vi "Coral Target Loop.vi"(0 "Camera Name":string="cam0") -> ()   [LabVIEW 2025]
uses:
  <vilib>/Utility/config.llb/NI_LVConfig.lvlib
  <vilib>/Utility/config.llb/Write Key (String).vi
  <vilib>/vision/NI_Vision_Development_Module.lvlib
  Camera Set Up/Event/Event Setup Types.ctl
  Ball/State Machine/Ball States.ctl
  <vilib>/Utility/config.llb/Read Key (String).vi
  Steam Type.ctl
  State Machine/Coral States.ctl
  <vilib>/vision/Image Controls.llb/IMAQ Image.ctl
  State Machine/Coral Main CLuster.ctl
  <vilib>/Rock Robotics/Network Tables/NT Write String.vi
  April Tags/Camera Info.ctl
panel:
  in  "Main":enum32{"Page 1", "Page 2"}(tab)
  out "Algae Distance":dbl[](array[numeric]) caption="Distance" format="%.1f"
  out "Algae Angle":dbl[](array[numeric]) caption="Angle" format="%.1f"
  out "Image":T1(plugin-control)
  in  "Settings":bool
  in  "Save":bool
  in  "Tools":bool
  out "Ball Fps":dbl format="%#.0f"
  in  "Robot Calibration Cluster":T2={"Camera FOV Vert View Angle (deg)"=34.5, "Camera FOV Hor View Angle (deg)"=28.3, "Distance Correction Factor"=0.946} {"Distance Correction Factor" format="%#_13g"; "Camera FOV Hor View Angle (deg)" format="%#_13g"; "Camera FOV Vert View Angle (deg)" format="%#_13g"}
  in  "Home":bool
  in  "Coral Color Range":T3={"Hue"={21.620689392089844, 69.62068939208984}, "Sat"={66.41378784179688, 255.0}, "Val"={96.0, 255.0}} caption="Color Range" {"Hue" scale=0.0..255.0 scale format="%#_3g"}
  out "Mask":T1(plugin-control)
  in  "Score Threshold %":dbl=80.0
  # "Edit the camera name to the camera that you are going to use for this target package"
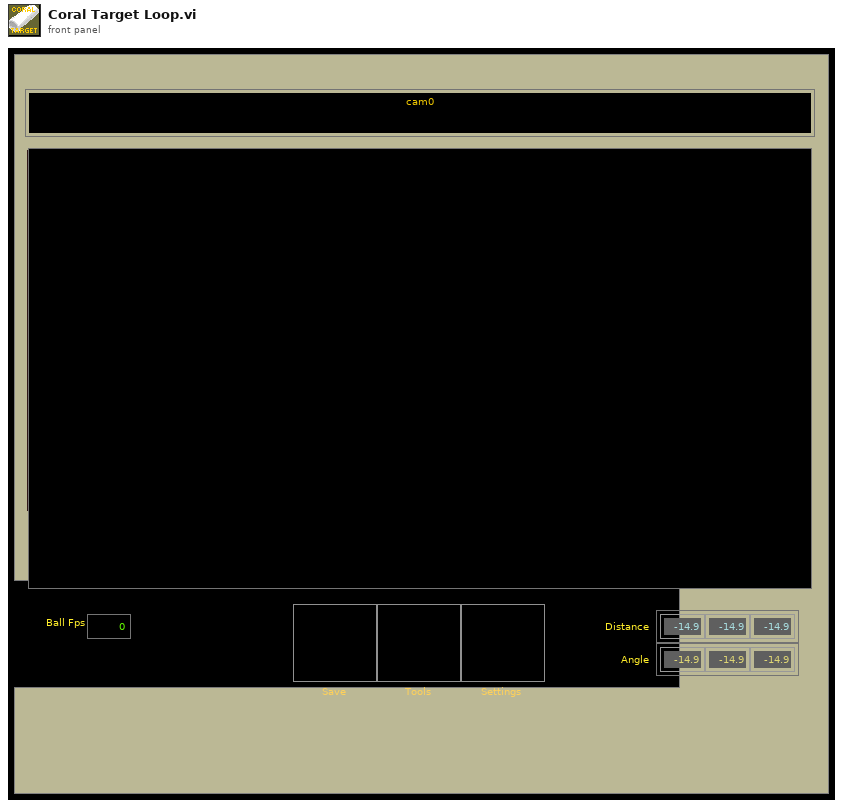
[diagram p1: front panel]
types:
  T1 = typedef "IMAQ Image.ctl" = refnum<image>
  T2 = typedef "Camera Info.ctl" = cluster{"Camera FOV Vert View Angle (deg)":dbl, "Camera FOV Hor View Angle (deg)":dbl, "Distance Correction Factor":dbl}
  T3 = cluster{"Hue":cluster{dbl, dbl}, "Sat":cluster{dbl, dbl}, "Val":cluster{dbl, dbl}}
  T4 = typedef "Coral Main CLuster.ctl" = cluster{"Coral FIFO":T5[], "Camera Name":string, "Coral path":path, "Control Ref's":refnum<vi>[], "Greyscale Mask Image":T1, "Main Image":T1, "Coral Color Range":cluster{"Hue":cluster{dbl, dbl}, "Sat":cluster{dbl, dbl}, "Val":cluster{dbl, dbl}}, "Timeout":i32}
  T5 = typedef "Coral States.ctl" = enum16{"Message Dispatcher", "INI", "Open", "Save", "Exit"}
  T6 = typedef "Particle Parameters" = i32
  T7 = typedef "Steam Type.ctl" = enum8{"Unknown", "Apriltag", "Algae", "Coral"}
  T8 = typedef "Event Setup Types.ctl" = enum16{"Default", "Camera Loop Started", "Close Settings", "GreyScale", "Open Front Panel", "Reset Team Number", "Save Data", "Exit"}
  T9 = typedef "Ball States.ctl" = enum16{"Message Dispatcher", "INI", "Open", "Save", "Exit"}
  T10 = typedef "Target Fields.ctl" = cluster{"diameter points":cluster{"first point":cluster{"x":dbl, "y":dbl}, "projected point":cluster{"x":dbl, "y":dbl}}, "normalized center":cluster{"x":dbl, "y":dbl}, "Overall Score":dbl, "Area Score":dbl, "Moment Score":dbl, "Aspect Score":dbl, "Distance (ft)":dbl, "Upper Goal":bool}
  T11 = typedef "Event Setup Types.ctl" = enum16{"Default", "Camera Loop Started", "GreyScale", "Reset Camera Settings", "Reset Team Number", "Save Data", "Setting Changed", "Update Video Mode", "Video Mode Changed", "Exit"}
  T12 = cluster{cluster{"Lower":dbl, "Upper":dbl}, cluster{"Lower":dbl, "Upper":dbl}, cluster{"Lower":dbl, "Upper":dbl}}
  T13 = typedef "Image Type" = u32
  T14 = typedef "NI_LVConfig.lvlib/Config Data RefNum.ctl" = refnum<k1>
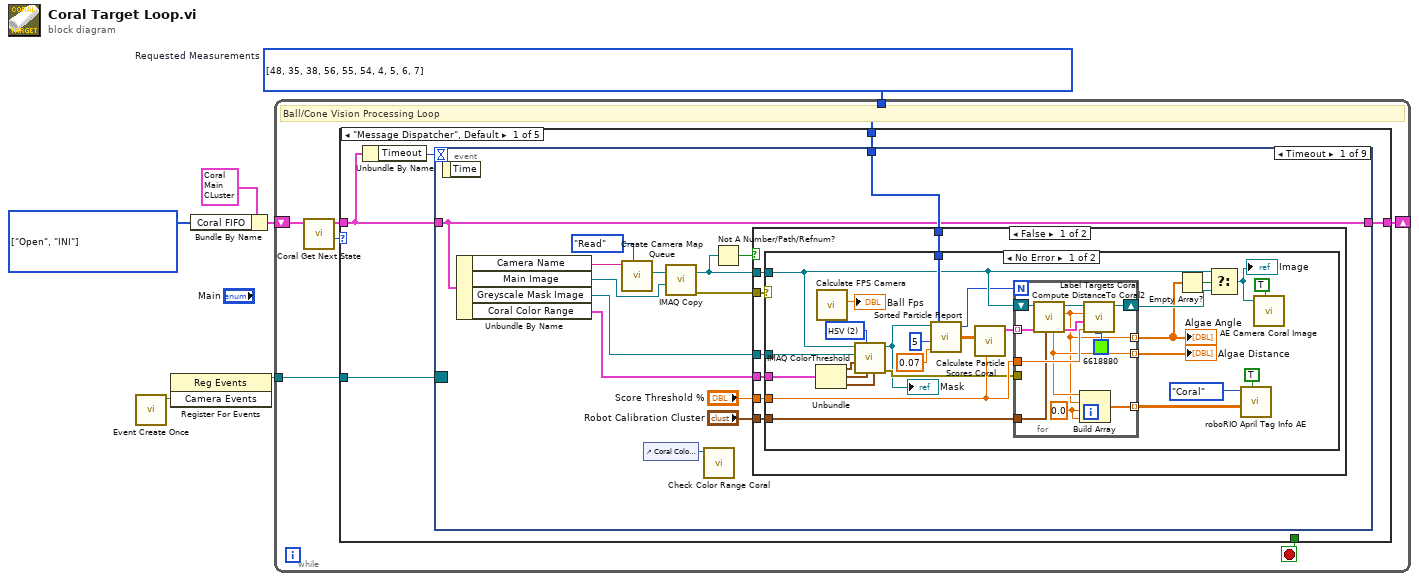
[diagram p0: block diagram]
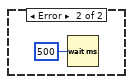
[diagram p2: hidden frame]
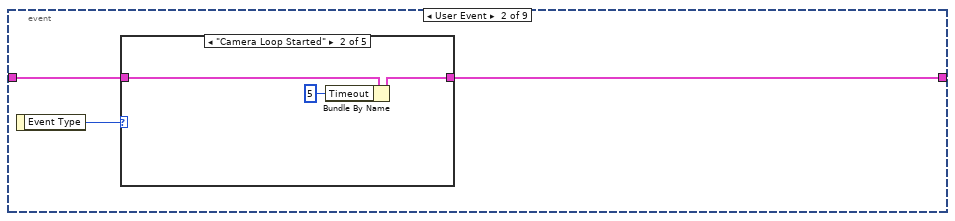
[diagram p4: hidden frame]
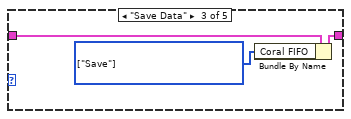
[diagram p6: hidden frame]
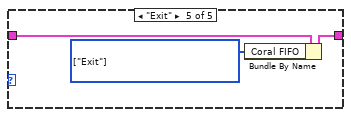
[diagram p8: hidden frame]
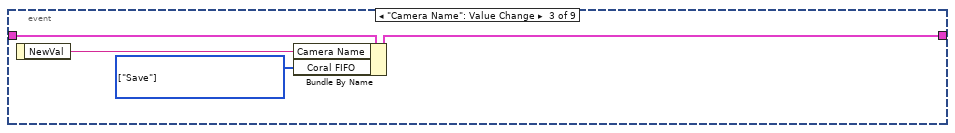
[diagram p9: hidden frame]
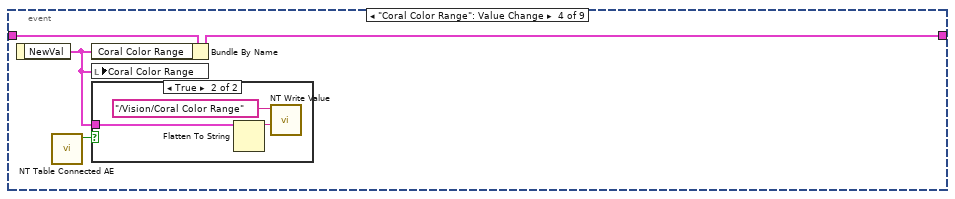
[diagram p10: hidden frame]
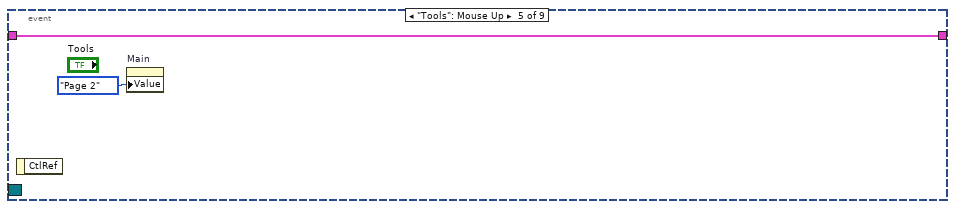
[diagram p12: hidden frame]
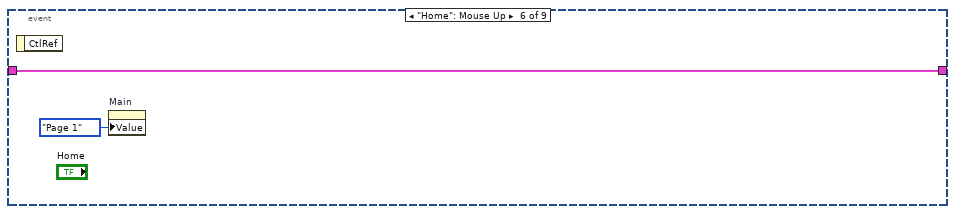
[diagram p13: hidden frame]
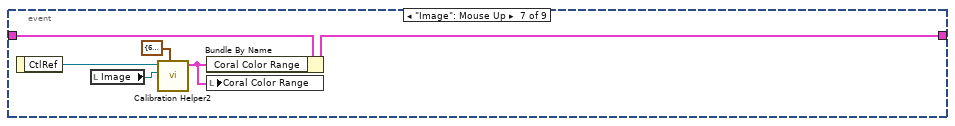
[diagram p14: hidden frame]
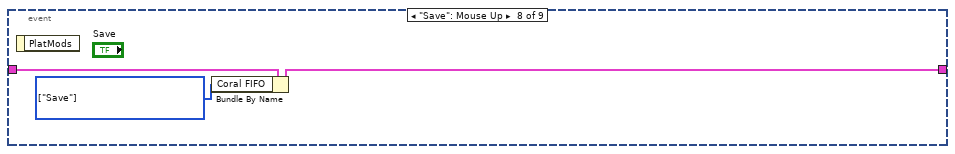
[diagram p15: hidden frame]
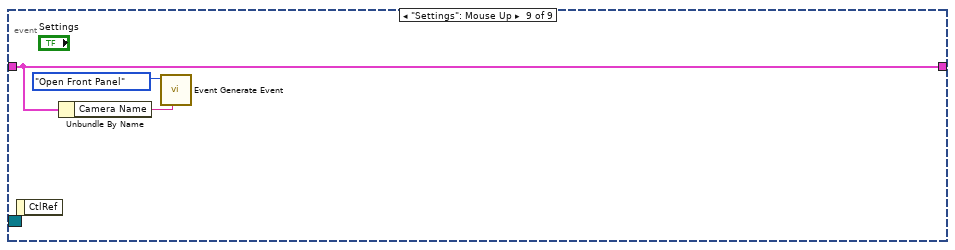
[diagram p16: hidden frame]
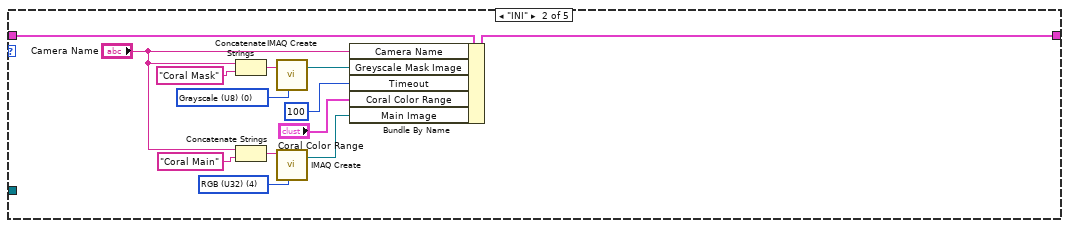
[diagram p17: hidden frame]
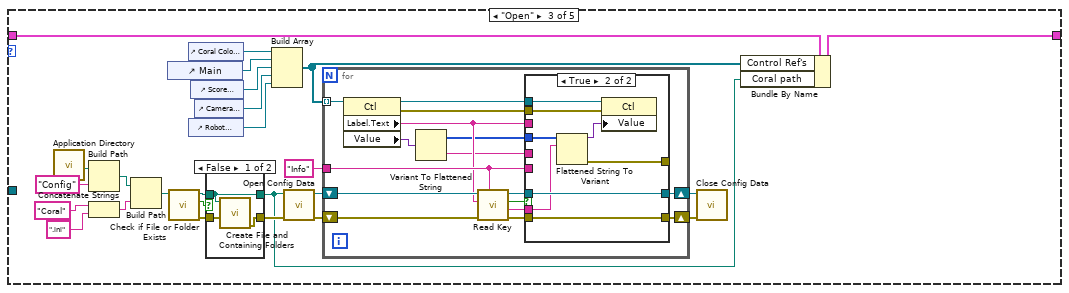
[diagram p18: hidden frame]
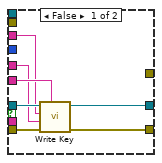
[diagram p20: hidden frame]
diagram:
  w2 = T5[] [enum."Open", enum."INI"] items=["Message Dispatcher", "INI", "Open", "Save", "Exit"] ("Ball FIFO")
  w4 = T6[] [48, 35, 38, 56, 55, 54, 4, 5, 6, 7] items=["Center of Mass X", "Center of Mass Y", "First Pixel X", "First Pixel Y", "Bounding Rect Left", "Bounding Rect Top", "Bounding Rect Right", "Bounding Rect Bottom", "Max Feret Diameter Start X", "Max Feret Diameter Start Y", "Max Feret Diameter End X", "Max Feret Diameter End Y", "Max Horiz. Segment Length Left", "Max Horiz. Segment Length Right", "Max Horiz. Segment Length Row", "-", "Bounding Rect Width", "Bounding Rect Height", "Bounding Rect Diagonal", "Perimeter", "Convex Hull Perimeter", "Holes' Perimeter", "Max Feret Diameter", "Equivalent Ellipse Major Axis", "Equivalent Ellipse Minor Axis", "Equivalent Ellipse Minor Axis (Feret)", "Equivalent Rect Long Side", "Equivalent Rect Short Side", "Equivalent Rect Diagonal", "Equivalent Rect Short Side (Feret)", "Average Horiz. Segment Length", "Average Vert. Segment Length", "Hydraulic Radius", "Waddel Disk Diameter", "-", "Area", "Holes' Area", "Particle & Holes' Area", "Convex Hull Area", "Image Area", "-", "Number of Holes", "Number of Horiz. Segments", "Number of Vert. Segments", "-", "Orientation", "Max Feret Diameter Orientation", "-", "% Area/Image Area", "% Area/(Particle & Holes' Area)", "Ratio of Equivalent Ellipse Axes", "Ratio of Equivalent Rect Sides", "-", "Elongation Factor", "Compactness Factor", "Heywood Circularity Factor", "Type Factor", "-", "Sum X", "Sum Y", "Sum XX", "Sum XY", "Sum YY", "Sum XXX", "Sum XXY", "Sum XYY", "Sum YYY", "-", "Moment of Inertia XX", "Moment of Inertia XY", "Moment of Inertia YY", "Moment of Inertia XXX", "Moment of Inertia XXY", "Moment of Inertia XYY", "Moment of Inertia YYY", "Norm. Moment of Inertia XX", "Norm. Moment of Inertia XY", "Norm. Moment of Inertia YY", "Norm. Moment of Inertia XXX", "Norm. Moment of Inertia XXY", "Norm. Moment of Inertia XYY", "Norm. Moment of Inertia YYY", "Hu Moment 1", "Hu Moment 2", "Hu Moment 3", "Hu Moment 4", "Hu Moment 5", "Hu Moment 6", "Hu Moment 7"]  # Requested Measurements
  n1 = call "Event Create Once.vi"() -> ("Camera Events"=w6:refnum<user-event>)  [unwired: 10 in, 1 out]
  n2 = register-events(w6) -> (reference out=w5:refnum<event-registration>)  [unwired: 2 in, 1 out]
  n3 = Bundle By Name(cluster=T4 {"Coral FIFO"=[], "Camera Name"="", "Coral path"=path "", "Control Ref's"=[], "Greyscale Mask Image"=refnum, "Main Image"=refnum, "Coral Color Range"={"Hue"={21.620689392089844, 69.62068939208984}, "Sat"={66.41378784179688, 255.0}, "Val"={96.0, 255.0}}, "Timeout"=5} ("output cluster"), "Coral FIFO"=w2) -> (w3:T4)
  n4 = while {
    tunnel: w4 -> [w13]
    tunnel: w5 -> [w12]
    shift-right: [w7] -> _
    shift-left: w3 -> [w10]
    stop <- w11 stop-if-true
    # "Ball/Cone Vision Processing Loop"
    n5 = call "Coral Get Next State.vi"("Coral Main Cluster in"=w10) -> ("Next State"=w9:T9, "Coral Main Cluster out"=w8:T4)  [unwired: 9 in]
    n6 = case shown="\"Message Dispatcher\", Default" w9 {
      tunnel: w13 -> [w18 _ _ _ _]
      tunnel: w12 -> [w17 _ _ _ _]
      tunnel: [_ _ _ _ TRUE] -> w11
      tunnel: w8 -> [w15 w130 w144 w197 w214]
      tunnel: [w16 w129 w142 w197 w214] -> w7
      frame "Message Dispatcher", Default {
        n7 = Unbundle By Name(w15) -> ("Timeout"=w14:i32)
        n8 = event shown="[0] Timeout" {
          selector: w17 -> [_ _ _ _ _ _ _ _ _]
          dyn-events: _ -> [_ _ _ _ _ _ _ _ _]
          timeout: w14 -> [_ _ _ _ _ _ _ _ _]
          tunnel: w18 -> [w32 _ _ _ _ _ _ _ _]
          tunnel: w15 -> [w27 w82 w97 w101 w105 w107 w111 w117 w119]
          tunnel: [w27 w80 w96 w100 w105 w107 w110 w116 w119] -> w16
          event Timeout {
            n9 = event-data() -> ()  [unwired: 1 in, 1 out]
            n10 = Unbundle By Name(w27) -> ("Camera Name"=w29:string, "Main Image"=w24:T1, "Greyscale Mask Image"=w28:T1, "Coral Color Range"=w26:T3)
            n11 = call "Create Camera Map Queue.vi"("Action"=enum16{"Read", "Write"}."Read", "Camera"=w29) -> ("Image out"=w25:T1)  [unwired: 8 in, 1 out]
            n12 = control-ref of="Coral Color Range"() -> (w21:refnum<vi>)
            n13 = call "IMAQ Copy"("Image Dst"=w24, "Image Src"=w25) -> ("error out"=w23:errorcluster, "Image Dst Out"=w19:T1)  [unwired: 4 in]
            n14 = call "Check Color Range Coral.vi"("Coral Color Range"=w21) -> ()  [unwired: 11 in]
            n15 = Not A Number/Path/Refnum?(number/path/refnum=w19) -> (NaN/Path/Refnum?=w20:bool)
            n16 = case shown="False" w20 {
              tunnel: w32 -> [w39 _]
              tunnel: "Score Threshold %" -> [w38 _]
              tunnel: w28 -> [w37 _]
              tunnel: w26 -> [w36 _]
              tunnel: w19 -> [w35 _]
              tunnel: w23 -> [w34 _]
              tunnel: "Robot Calibration Cluster" -> [w33 _]
              frame False {
                n17 = case shown="No Error" w34 {
                  tunnel: w39 -> [w66 _]
                  tunnel: w37 -> [w64 _]
                  tunnel: w36 -> [w63 _]
                  tunnel: w38 -> [w62 _]
                  tunnel: w35 -> [w61 _]
                  tunnel: w33 -> [w41 _]
                  frame No Error {
                    w56 = u16 2 items=["RGB", "HSL", "HSV", "HSI"] ("Color Mode")
                    n18 = Unbundle(w63) -> ("Hue"=w51:cluster{dbl, dbl}, "Sat"=w50:cluster{dbl, dbl}, "Val"=w49:cluster{dbl, dbl})
                    n19 = call "Calculate FPS Camera.vi"() -> ("Fps"=→"Ball Fps":dbl)  [unwired: 11 in]
                    n20 = call "IMAQ ColorThreshold"("Blue or Luma or Val or Inten Range"=w49, "Green or Sat Range"=w50, "Color Mode"=w56, "Red or Hue Range"=w51, "Image Dst"=w64, "Image Src"=w61) -> ("error out"=w55:errorcluster, "Image Dst Out"=w40:T1)  [unwired: 4 in]
                    "Mask" <- w40
                    n21 = call "Sorted Particle Report.vi"("Min Area Size %"=0.07 ("Size Limit %"), "Particle Count Limit"=5 ("Particle Count LImit"), "Pixel Measurements"=w66, "Image in"=w40) -> ("Sorted Data"=w59:dbl[][], "Particles"=w54:i32)  [unwired: 1 out]
                    n22 = call "Calculate Particle Scores Coral.vi"("Limit"=w62, "Sorted Data"=w59) -> ("Scores"=w58:T10[])  [unwired: 9 in]
                    n23 = for {
                      N: w54 -> [_]
                      tunnel: w58 -> [w76] mode=indexing
                      shift-right: [w78] -> w53
                      shift-left: w61 -> [w74]
                      tunnel: w62 -> [w77]
                      tunnel: [w70] -> w48 mode=indexing
                      tunnel: w55 -> [_]
                      tunnel: [w71] -> w47 mode=indexing
                      tunnel: [w68] -> w42 mode=indexing
                      tunnel: w41 -> [w67]
                      w69 = 0.0 ("element")
                      n24 = call "Compute DistanceTo Coral2.vi"("Robot Calibration Cluster"=w67, "results 2"=w76, "Image Src"=w74) -> ("results out"=w73:T10, "Offset Angle"=w70:dbl, "Image Dst Out"=w75:T1, "Distance from target (in)"=w71:dbl)  [unwired: 5 in]
                      n25 = Build Array(w71, w70, w69, w69) -> (w68:dbl[])
                      n26 = call "Label Targets Coral.vi"("Color"=u32 6618880, "Score Threshold"=w77, "results"=w73, "Angle"=w70, "Image in"=w75) -> ("Image out"=w78:T1)  [unwired: 6 in]
                    }
                    "Algae Angle" <- w48
                    "Algae Distance" <- w47
                    n27 = Empty Array?(array=w48) -> (empty?=w52:bool)
                    n28 = Select(t=w61, s=w52, f=w53) -> (s? t:f=w65:T1)
                    "Image" <- w65
                    n29 = call "roboRIO April Tag Info AE.vi"("Update"=TRUE, "Info in"=w42, "Stream Type"=Steam_Type."Coral") -> ()  [unwired: 8 in, 1 out]
                    n30 = call "AE Camera Coral Image.vi"("Update"=TRUE, "Ball Image in"=w65) -> ()  [unwired: 9 in, 1 out]
                  }
                  frame Error {
                    n31 = Wait (ms)(milliseconds to wait=u32 500) -> ()  [unwired: 1 out]
                  }
                }
              }
              frame True {
              }
            }
          }
          event User Event {
            n32 = event-data() -> ("Event Type"=w81:T11)  [unwired: 1 in]
            n33 = case shown="\"Camera Loop Started\"" w81 {
              tunnel: w82 -> [w83 w86 w89 w90 w93]
              tunnel: [w83 w85 w88 w90 w92] -> w80
              frame "Default", Default {
              }
              frame "Camera Loop Started" {
                n34 = Bundle By Name(cluster=w86, "Timeout"=5) -> (w85:T4)
              }
              frame "Save Data" {
                w87 = T9[] [enum."Save"] items=["Message Dispatcher", "INI", "Open", "Save", "Exit"] ("Ball FIFO")
                n35 = Bundle By Name(cluster=w89, "Coral FIFO"=w87) -> (w88:T4)
              }
              frame "Default" {
              }
              frame "Exit" {
                w91 = T9[] [enum."Exit"] items=["Message Dispatcher", "INI", "Open", "Save", "Exit"] ("Ball FIFO")
                n36 = Bundle By Name(cluster=w93, "Coral FIFO"=w91) -> (w92:T4)
              }
            }
          }
          event "Camera Name": Value Change {
            w94 = T9[] [enum."Save"] items=["Message Dispatcher", "INI", "Open", "Save", "Exit"] ("Ball FIFO")
            n37 = event-data() -> ("NewVal"=w95:string)  [unwired: 1 in]
            n38 = Bundle By Name(cluster=w97, "Camera Name"=w95, "Coral FIFO"=w94) -> (w96:T4)
          }
          event "Coral Color Range": Value Change {
            n39 = event-data() -> ("NewVal"=w98:T3)  [unwired: 1 in]
            n40 = call "NT Table Connected AE.vi"() -> ("NT Table Connected out"=w99:bool)  [unwired: 11 in]
            n41 = Bundle By Name(cluster=w101, "Coral Color Range"=w98) -> (w100:T4)
            n42 = local write "Coral Color Range"(w98) -> ()
            n43 = case shown="True" w99 {
              tunnel: w98 -> [_ w102]
              frame False {
              }
              frame True {
                n44 = Flatten To String(anything=w102) -> (data string=w104:string)  [unwired: 3 in, 2 out]
                n45 = call-poly <vilib>:"NT Write Value.vi"("value"=w104, "name"="/Vision/Coral Color Range" ("Name")) -> ()  [unwired: 9 in, 1 out]
              }
            }
          }
          event "Tools": Mouse Up {
            n46 = event-data() -> ()  [unwired: 1 in, 1 out]
            n47 = property on="Main" class="TabCtl (strict)"("Value"=enum32{"Page 1", "Page 2"}."Page 2" ("Main")) -> ()  [unwired: 2 in, 2 out]
          }
          event "Home": Mouse Up {
            n48 = event-data() -> ()  [unwired: 1 in, 1 out]
            n49 = property on="Main" class="TabCtl (strict)"("Value"=enum32{"Page 1", "Page 2"}."Page 1" ("Main")) -> ()  [unwired: 2 in, 2 out]
          }
          event "Image": Mouse Up {
            n50 = event-data() -> ("CtlRef"=w113:refnum<vi>)  [unwired: 1 in]
            n51 = local read "Image"() -> (w112:T1)
            n52 = call "Calibration Helper2.vi"("Std Devs"=cluster{"H":dbl, "S":dbl, "V":dbl} {"H"=6.0, "S"=6.0, "V"=6.0} ("Std Devs Ball"), "Image"=w112, "Image Ctl Refnum"=w113) -> ("output color"=w109:T12)  [unwired: 7 in, 1 out]
            n53 = Bundle By Name(cluster=w111, "Coral Color Range"=w109) -> (w110:T4)
            n54 = local write "Coral Color Range"(w109) -> ()
          }
          event "Save": Mouse Up {
            w115 = T9[] [enum."Save"] items=["Message Dispatcher", "INI", "Open", "Save", "Exit"] ("Ball FIFO")
            n55 = event-data() -> ()  [unwired: 1 in, 1 out]
            n56 = Bundle By Name(cluster=w117, "Coral FIFO"=w115) -> (w116:T4)
          }
          event "Settings": Mouse Up {
            n57 = event-data() -> ()  [unwired: 1 in, 1 out]
            n58 = Unbundle By Name(w119) -> ("Camera Name"=w118:string)
            n59 = call "Event Generate Event.vi"("Camera Name"=w118, "Event Type"=Event_Setup_Types."Open Front Panel") -> ()  [unwired: 10 in]
          }
        }
      }
      frame "INI" {
        w126 = T13 4 items=["Grayscale (U8)", "Grayscale (I16)", "Grayscale (SGL)", "Complex (CSG)", "RGB (U32)", "HSL (U32)", "RGB (U64)", "Grayscale (U16)"] ("Image Type")
        w131 = T13 0 items=["Grayscale (U8)", "Grayscale (I16)", "Grayscale (SGL)", "Complex (CSG)", "RGB (U32)", "HSL (U32)", "RGB (U64)", "Grayscale (U16)"] ("Image Type")
        n60 = Concatenate Strings("Camera Name", "Coral Mask" ("string")) -> (w133:string)
        n61 = Concatenate Strings("Camera Name", "Coral Main" ("string")) -> (w125:string)
        n62 = call "IMAQ Create"("Image Name"=w133, "Image Type"=w131) -> ("New Image"=w128:T1)  [unwired: 2 in, 2 out]
        n63 = call "IMAQ Create"("Image Name"=w125, "Image Type"=w126) -> ("New Image"=w122:T1)  [unwired: 2 in, 2 out]
        n64 = Bundle By Name(cluster=w130, "Camera Name"="Camera Name", "Greyscale Mask Image"=w128, "Timeout"=100, "Coral Color Range"="Coral Color Range", "Main Image"=w122) -> (w129:T4)
      }
      frame "Open" {
        n65 = call <vilib>:"Application Directory.vi"() -> ("Application Directory"=w147:path)
        n66 = Build Path(base path=w147, name or relative path="Config") -> (appended path=w145:path)
        n67 = Concatenate Strings("Coral" ("string"), ".ini" ("name or relative path")) -> (w158:string)
        n68 = Build Path(base path=w145, name or relative path=w158) -> (appended path=w140:path)
        n69 = control-ref of="Main"() -> (w151:refnum<vi>)
        n70 = call <vilib>:"Check if File or Folder Exists.vi"("path"=w140) -> ("error out"=w136:errorcluster, "file or folder exists?"=w138:bool, "dup path"=w139:path)  [unwired: 8 in]
        n71 = control-ref of="Coral Color Range"() -> (w152:refnum<vi>)
        n72 = control-ref of="Robot Calibration Cluster"() -> (w134:refnum<vi>)
        n73 = control-ref of="Score Threshold %"() -> (w150:refnum<vi>)
        n74 = control-ref of="Camera Name"() -> (w135:refnum<vi>)
        n75 = case shown="False" w138 {
          tunnel: [w161 w162] -> w148
          tunnel: w139 -> [w160 w163]
          tunnel: [w160 w163] -> w137
          tunnel: w136 -> [w159 w162]
          frame False {
            n76 = call <vilib>:"Create File and Containing Folders.vi"("error in (no error)"=w159, "file path"=w160) -> ("error out"=w161:errorcluster)  [unwired: 8 in, 1 out]
          }
          frame True {
          }
        }
        n77 = Build Array(w152, w151, w150, w135, w134) -> (w141:refnum<vi>[])
        n78 = call <vilib>:"Open Config Data.vi"("error in (no error)"=w148, "configuration file path"=w137) -> ("error out"=w153:errorcluster, "refnum"=w157:T14)  [unwired: 7 in, 1 out]
        n79 = for {
          tunnel: "Info" ("Camera Name") -> [w176]
          tunnel: w141 -> [w166] mode=indexing
          shift-right: [w178] -> w156
          shift-left: w157 -> [w179]
          shift-right: [w177] -> w155
          shift-left: w153 -> [w175]
          n80 = property class="Ctl"(reference=w166) -> (reference out=w172:refnum<vi>, error out=w171:errorcluster, "Label.Text"=w169:string, "Value"=w165:variant)  [unwired: 1 in]
          n81 = Variant To Flattened String(Variant=w165) -> (data string=w167:string, 1:w164:i16[])
          n82 = call-poly <vilib>:"Read Key.vi"("section"=w176, "error in (no error)"=w175, "key"=w169, "refnum"=w179) -> ("error out"=w168:errorcluster, "value"=w173:string, "found?"=w174:bool, "refnum out"=w170:T14)  [unwired: 4 in]
          n83 = case shown="True" w174 {
            tunnel: w173 -> [_ w189]
            tunnel: w172 -> [_ w194]
            tunnel: w171 -> [_ w193]
            tunnel: w170 -> [w186 w192]
            tunnel: w176 -> [w185 _]
            tunnel: w169 -> [w184 _]
            tunnel: [w183 w192] -> w178
            tunnel: w168 -> [w182 w191]
            tunnel: [w181 w191] -> w177
            tunnel: w167 -> [w180 _]
            tunnel: w164 -> [_ w188]
            tunnel: [_ w187] -> _
            frame False {
              n84 = call-poly <vilib>:"Write Key.vi"("section"=w185, "error in (no error)"=w182, "value"=w180, "key"=w184, "refnum"=w186) -> ("error out"=w181:errorcluster, "refnum out"=w183:T14)  [unwired: 4 in, 1 out]
            }
            frame True {
              n85 = Flattened String To Variant(6:w189, 7:w188) -> (0:w187:errorcluster, 3:w190:variant)  [unwired: 1 in]
              n86 = property class="Ctl"(reference=w194, error in=w193, "Value"=w190) -> ()  [unwired: 2 out]
            }
          }
        }
        n87 = call <vilib>:"Close Config Data.vi"("error in (no error)"=w155, "refnum"=w156) -> ()  [unwired: 8 in, 2 out]
        n88 = Bundle By Name(cluster=w144, "Control Ref's"=w141, "Coral path"=w137) -> (w142:T4)
      }
      frame "Save" {
        n89 = Unbundle By Name(w197) -> ("Control Ref's"=w195:refnum<vi>[], "Coral path"=w196:path)
        n90 = call <vilib>:"Open Config Data.vi"("configuration file path"=w196) -> ("error out"=w201:errorcluster, "refnum"=w202:T14)  [unwired: 8 in, 1 out]
        n91 = for {
          tunnel: w195 -> [w212] mode=indexing
          tunnel: w202 -> [w211]
          tunnel: w201 -> [w210]
          tunnel: "Info" ("Camera Name") -> [w206]
          tunnel: [w204] -> w200
          tunnel: [w203] -> w199
          n92 = property class="Ctl"(reference=w212, error in=w210) -> (error out=w207:errorcluster, "Label.Text"=w209:string, "Value"=w208:variant)  [unwired: 1 out]
          n93 = Variant To Flattened String(Variant=w208) -> (data string=w205:string)  [unwired: 1 out]
          n94 = call-poly <vilib>:"Write Key.vi"("section"=w206, "error in (no error)"=w207, "value"=w205, "key"=w209, "refnum"=w211) -> ("error out"=w204:errorcluster, "refnum out"=w203:T14)  [unwired: 4 in, 1 out]
        }
        n95 = call <vilib>:"Close Config Data.vi"("error in (no error)"=w200, "refnum"=w199) -> ()  [unwired: 8 in, 2 out]
      }
      frame "Exit" {
        n96 = Unbundle By Name(w214) -> ("Greyscale Mask Image"=w216:T1, "Main Image"=w215:T1)
        n97 = call "IMAQ Dispose"("Image"=w216) -> ()  [unwired: 5 in, 1 out]
        n98 = call "IMAQ Dispose"("Image"=w215) -> ()  [unwired: 5 in, 1 out]
      }
    }
  }
